vi "Connect Sensor.vi"(8 "error in (no error)":errorcluster, 9 "lpszDataPath":string, 10 "nSensorIP":u32, 11 "nHostIP":u32) -> (0 "error out":errorcluster, 1 "lpszDataPath out":string, 3 "Return Code":u16(ring) items=["IMAGECAP_OK"=0, "IMAGECAP_SOCKET_LOAD_ERROR"=1, "IMAGECAP_INVALID_SOCKET_ERROR"=2, "IMAGECAP_BIND_SOCKET_ERROR"=3, "IMAGECAP_SOCKET_OPTION_ERROR"=4, "IMAGECAP_COMMAND_SEND_ERROR"=5, "IMAGECAP_COMMAND_RECV_ERROR"=6, "IMAGECAP_RECV_TIMEOUT_ERROR"=7, "IMAGECAP_ACK_SEND_ERROR"=8, "IMAGECAP_NO_SENSOR_ERROR"=9, "IMAGECAP_REGISTER_TYPE_ERROR"=10, "IMAGECAP_GET_HOST_NAME_ERROR"=11, "IMAGECAP_NIC_CHECK"=12, "IMAGECAP_STOP_WAIT"=13, "IMAGECAP_CANCEL"=16, "IMAGECAP_NEW_FRAME"=256, "IMAGECAP_RECEIVING"=257, "IMAGECAP_NOTREADY_RO"=272, "IMAGECAP_NOTSUPPORTED"=273])   [LabVIEW 2017, in "imgAcquisition.lvlib"]
doc: "DLLFunction int __stdcall ImageCapConnectSensor(unsigned int nHostIP, unsigned int nSensorIP, LPCTSTR lpszDataPath);"
uses:
  imgAcquisition.lvlib
  lib/ImageCaptureDLL.dll
panel:
  out "function return":u16 format="%x"
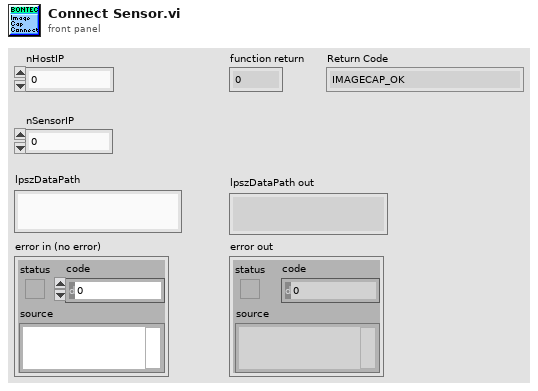
[diagram p1: front panel]
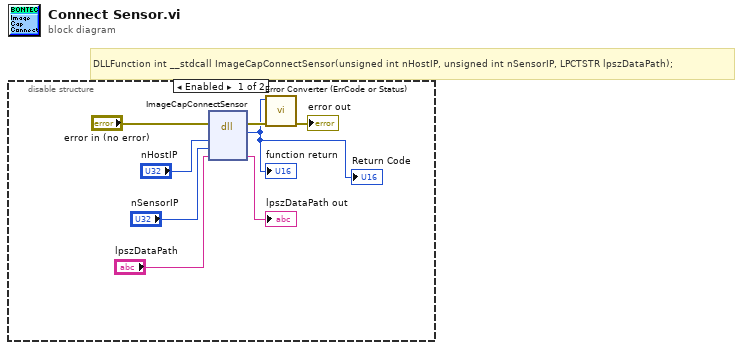
[diagram p0: block diagram]
diagram:
  # "DLLFunction int __stdcall ImageCapConnectSensor(unsigned int nHostIP, unsigned int nSensorIP, LPCTSTR lpszDataPath);"
  n1 = disable-structure shown="Enabled" {
    frame Enabled {
      n2 = dll-call lib="F:/BonTechFlatPanelLVDriver/lib/ImageCaptureDLL.*" fn="ImageCapConnectSensor"(error in="error in (no error)", "nHostIP"="nHostIP", "nSensorIP"="nSensorIP", "lpszDataPath"="lpszDataPath") -> (error out=w3:errorcluster, w1:i32, "lpszDataPath"=→"lpszDataPath out":string)  [unwired: 4 in, 1 out]
      "function return" <- w1
      "Return Code" <- w1
      n3 = call "Error Converter (ErrCode or Status).vi"("error in (no error)"=w3, "error code"=w1) -> ("error out"=→"error out":errorcluster)  [unwired: 9 in]
    }
    frame Disabled {
    }
  }
